vi "Enumerate cameras.vi"() -> (0 "Error Out":errorcluster, 1 "Camera Information Array":T1(array[cluster]) {"BusType" format="%x"; "SerialNumberLow" format="%.0x"; "SerialNumberHigh" format="%.0x"})   [LabVIEW 2014]
uses:
  <vilib>/vision/driver/NI_Vision_Acquisition_Software.lvlib
panel:
  # "PN 27/11/2014"
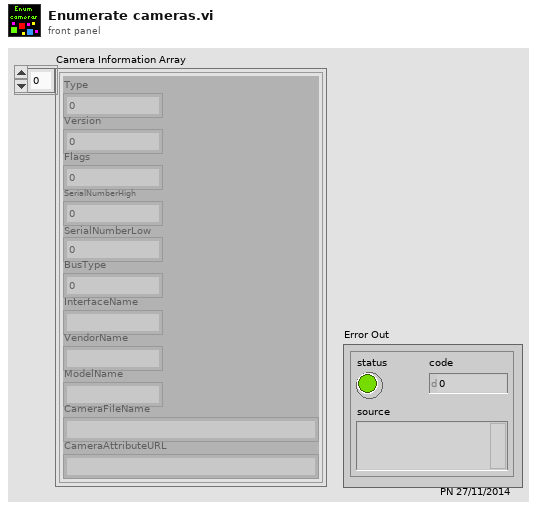
[diagram p1: front panel]
types:
  T1 = cluster{"Type":u32, "Version":u32, "Flags":u32, "SerialNumberHigh":u32, "SerialNumberLow":u32, "BusType":u32, "InterfaceName":string, "VendorName":string, "ModelName":string, "CameraFileName":string, "CameraAttributeURL":string}[]
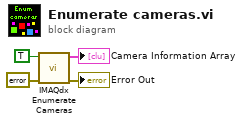
[diagram p0: block diagram]
diagram:
  n1 = call <vilib>:"IMAQdx Enumerate Cameras.vi"("error in"=errorcluster {"status"=FALSE, "code"=0, "source"=""}, "Connected Only? (Yes)"=TRUE) -> ("error out"=→"Error Out":errorcluster, "Camera Information Array"=→"Camera Information Array":T1)  [unwired: 8 in]
